vi "Create Evaluations.vi"(8 "error in (no error)":errorcluster, 11 "TDSCDMA_SEM in":refnum<class "TDSCDMA_SEM.lvclass">) -> (0 "error out":errorcluster, 2 "Evaluations Out":T1[](array[typedef]) {"Low Limit" format="%#_13g"; "SI Scaling" items=["femto"=-15, "pico"=-12, "nano"=-9, "micro"=-6, "milli"=-3, "percent"=-2, ""=0, "kilo"=3, "mega"=6, "giga"=9, "tera"=12]}, 3 "TDSCDMA_SEM out":refnum<class "TDSCDMA_SEM.lvclass">)   [LabVIEW 2016, in "SeqAuto Evaluations.lvlib" / "TDSCDMA_SEM.lvclass"]
uses:
  TDSCDMA_SEM.lvclass
  C:/projects/STS/Common/Sequence Automation/Plugins/SeqAuto IEvaluation.lvlibp/SeqAuto IEvaluation.lvclass
  Plugins/TestStand API Tools (TSAT).lvlibp/Evaluation Actions/Includes/Controls/TSAT Evaluation.ctl
  Plugins/TestStand API Tools (TSAT).lvlibp/Evaluation Actions/Includes/Controls/TSAT Eval SI Unit Scaling.ctl
  Plugins/TestStand API Tools (TSAT).lvlibp/Evaluation Actions/Includes/Controls/TSAT Evaluation Type.ctl
  Plugins/SeqAuto IEvaluation.lvlibp/Read Measurement Name.vi
  Plugins/TestStand API Tools (TSAT).lvlibp/Evaluation Actions/TSAT Evaluation Actions.lvlib
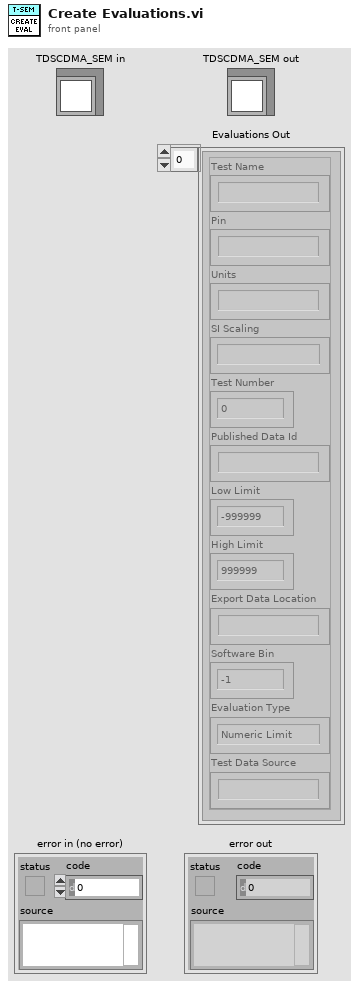
[diagram p1: front panel]
types:
  T1 = typedef "TestStand API Tools (TSAT).lvlibp/TSAT Evaluation Actions.lvlib/TSAT Evaluation.ctl" = cluster{"Test Name":string, "Pin":string, "Units":string, "SI Scaling":T2, "Test Number":i32, "Published Data Id":string, "Low Limit":dbl, "High Limit":dbl, "Export Data Location":string, "Software Bin":i64, "Evaluation Type":T3, "Test Data Source":string}
  T2 = typedef "TestStand API Tools (TSAT).lvlibp/TSAT Evaluation Actions.lvlib/TSAT Eval SI Unit Scaling.ctl" = i16
  T3 = typedef "TestStand API Tools (TSAT).lvlibp/TSAT Evaluation Actions.lvlib/TSAT Evaluation Type.ctl" = enum16{"Numeric Limit", "Pass/Fail", "None"}
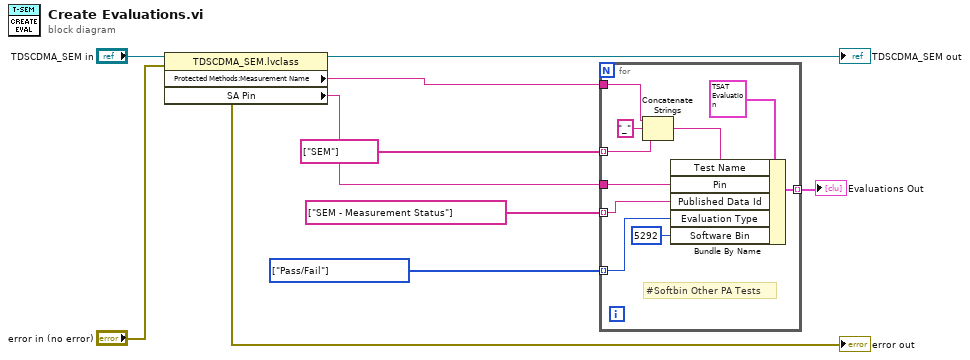
[diagram p0: block diagram]
diagram:
  w4 = T3[] [enum."Pass/Fail"] items=["Numeric Limit", "Pass/Fail", "None"]
  n1 = property class="TDSCDMA_SEM.lvclass"(reference="TDSCDMA_SEM in", error in="error in (no error)") -> (reference out=→"TDSCDMA_SEM out":refnum<class "TDSCDMA_SEM.lvclass">, error out=→"error out":errorcluster, "Protected Methods:Measurement Name"=w2:string, "SA Pin"=w1:string)
  n2 = for {
    tunnel: string[] ["SEM"] -> [w19] mode=indexing
    tunnel: string[] ["SEM - Measurement Status"] -> [w16] mode=indexing
    tunnel: w4 -> [w15] mode=indexing
    tunnel: [w14] -> w3 mode=indexing
    tunnel: w2 -> [w13]
    tunnel: w1 -> [w12]
    # "#Softbin Other PA Tests"
    n3 = Concatenate Strings(w13, "_" ("string"), w19) -> (w18:string)
    n4 = Bundle By Name(cluster=T1 {"Test Name"="", "Pin"="", "Units"="", "SI Scaling"=0, "Test Number"=0, "Published Data Id"="", "Low Limit"=-999999.0, "High Limit"=999999.0, "Export Data Location"="", "Software Bin"=-1, "Evaluation Type"=enum."Numeric Limit", "Test Data Source"=""} ("Evaluation"), "Test Name"=w18, "Pin"=w12, "Published Data Id"=w16, "Evaluation Type"=w15, "Software Bin"=i64 5292) -> (w14:T1)
  }
  "Evaluations Out" <- w3
